vi "Get Manipulator Shoot Location.vi"(10 "Manipulator Buttons":T2, 11 "Manipulator Axes":T3) -> (0 "Manual Buttons":T1, 3 "Shoot Location":T4, 5 "Location Selected":bool)   [LabVIEW 2013]
uses:
  Shoot Location.ctl
  <vilib>/Rock Robotics/WPI/Joystick/WPI_JoystickButtonState.ctl
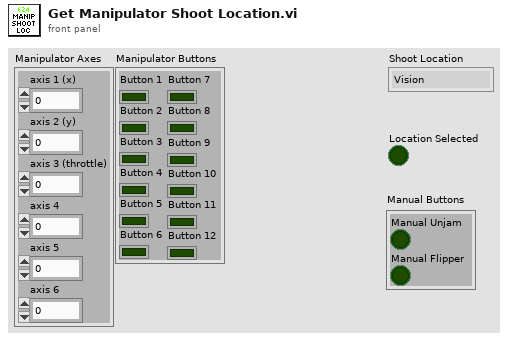
[diagram p1: front panel]
types:
  T1 = cluster{"Manual Unjam":bool, "Manual Flipper":bool}
  T2 = typedef "WPI_JoystickButtonState.ctl" = cluster{"Button 1":bool, "Button 2":bool, "Button 3":bool, "Button 4":bool, "Button 5":bool, "Button 6":bool, "Button 7":bool, "Button 8":bool, "Button 9":bool, "Button 10":bool, "Button 11":bool, "Button 12":bool}
  T3 = cluster{"axis 1 (x)":dbl, "axis 2 (y)":dbl, "axis 3 (throttle)":dbl, "axis 4":dbl, "axis 5":dbl, "axis 6":dbl}
  T4 = typedef "Shoot Location.ctl" = enum16{"Vision", "Front", "Front Corner", "Back Corner", "Half Court", "Full Court", "Pyramid"}
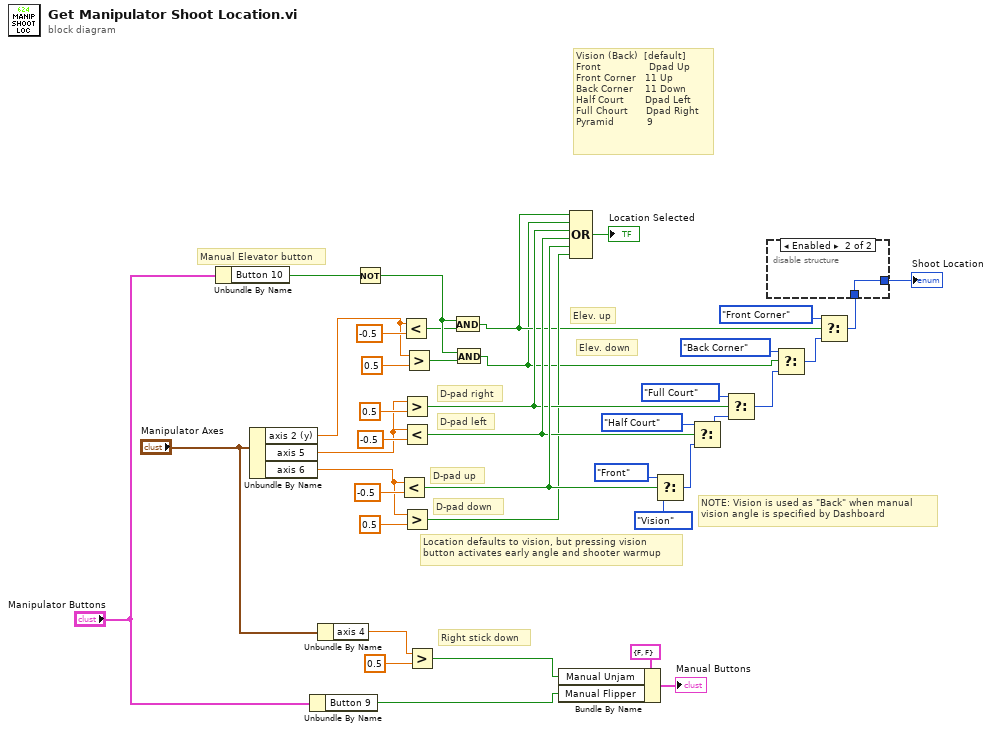
[diagram p0: block diagram]
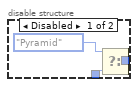
[diagram p2: hidden frame]
diagram:
  # "Right stick down"
  # "Manual Elevator button"
  # "NOTE: Vision is used as \"Back\" when manual\nvision angle is specified by Dashboard"
  # "Location defaults to vision, but pressing vision\nbutton activates early angle and shooter warmup"
  # "Vision (Back)  [default]\nFront               \tDpad Up\nFront Corner  \t11 Up\nBack Corner\t   11 Down\nHalf Court      \tDpad Left\nFull Chourt     \tDpad Right\nPyramid\t          9"
  # "Elev. up"
  # "Elev. down"
  # "D-pad up"
  # "D-pad down"
  # "D-pad left"
  # "D-pad right"
  n1 = Unbundle By Name("Manipulator Buttons") -> ("Button 10"=w14:bool)
  n2 = Unbundle By Name("Manipulator Axes") -> ("axis 2 (y)"=w32:dbl, "axis 5"=w38:dbl, "axis 6"=w35:dbl)
  n3 = Unbundle By Name("Manipulator Buttons") -> ("Button 9"=w1:bool)
  n4 = Unbundle By Name("Manipulator Axes") -> ("axis 4"=w5:dbl)
  n5 = Not(x=w14) -> (.not. x?=w13:bool)
  n6 = Less?(x=w35, y=-0.5) -> (x < y?=w19:bool)
  n7 = Less?(x=w32, y=-0.5) -> (x < y?=w12:bool)
  n8 = Greater?(x=w38, y=0.5) -> (0:w17:bool)
  n9 = Less?(x=w38, y=-0.5) -> (x < y?=w18:bool)
  n10 = Greater?(x=w35, y=0.5) -> (0:w15:bool)
  n11 = Greater?(x=w32, y=0.5) -> (0:w10:bool)
  n12 = Greater?(x=w5, y=0.5) -> (0:w2:bool)
  n13 = And(x=w13, y=w12) -> (x .and. y?=w11:bool)
  n14 = And(x=w13, y=w10) -> (x .and. y?=w9:bool)
  n15 = Bundle By Name(cluster=T1 {"Manual Unjam"=FALSE, "Manual Flipper"=FALSE} ("Manual Buttons"), "Manual Unjam"=w2, "Manual Flipper"=w1) -> (→"Manual Buttons":T1)
  n16 = Compound Arithmetic op=OR(w11, w9, w17, w18, w19, w15) -> (→"Location Selected":bool)
  n17 = Select(t=Shoot_Location."Front", s=w19, f=Shoot_Location."Vision" ("Shoot Location")) -> (s? t:f=w29:T4)
  n18 = Select(t=Shoot_Location."Half Court", s=w18, f=w29) -> (s? t:f=w31:T4)
  n19 = Select(t=Shoot_Location."Full Court", s=w17, f=w31) -> (s? t:f=w28:T4)
  n20 = Select(t=Shoot_Location."Back Corner", s=w9, f=w28) -> (s? t:f=w30:T4)
  n21 = Select(t=Shoot_Location."Front Corner", s=w11, f=w30) -> (s? t:f=w21:T4)
  n22 = disable-structure shown="Enabled" {
    disable-tunnel: w21 -> [w44 w45]
    disable-tunnel: [w42 w45] -> w20
    frame Disabled {
      n23 = Select(t=Shoot_Location."Pyramid" ("Shoot Location"), f=w44) -> (s=w41:bool, s? t:f=w42:T4)
    }
    frame Enabled {
    }
  }
  "Shoot Location" <- w20
